vi "MCCMSG Select Multi Clamp.vi"(0 "hMCCmsg":i32, 1 "uDeviceID":u32, 2 "pnError":i32, 5 "uModel":u32, 7 "pszSerialNum":string, 9 "uCOMPortID":u32, 11 "error in (no error)":errorcluster, 12 "uChannelID":u32) -> (4 "pnError out":i32, 6 "function return":i32, 8 "pszSerialNum out":string, 15 "error out":errorcluster)   [LabVIEW 2012, in "MultiClamp 700B Controls.lvlib" / "AxMultiClampMsg.lvlib"]
doc: "AXMCCMSG BOOL WINAPI MCCMSG_SelectMultiClamp(HMCCMSG hMCCmsg, UINT uModel, char *pszSerialNum, UINT uCOMPortID, UINT uDeviceID, UINT uChannelID, int *pnError);"
uses:
  AxMultiClampMsg.lvlib
  AxMultiClampMsg.dll
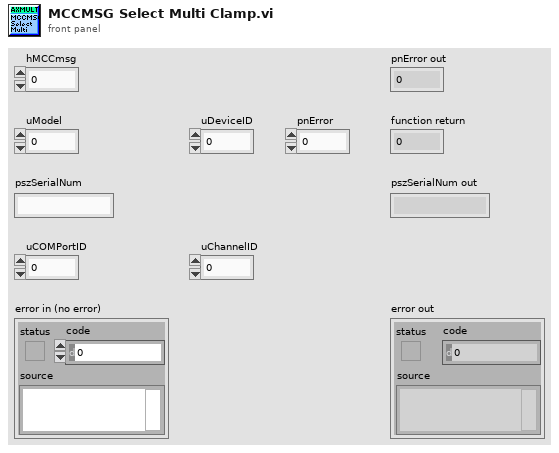
[diagram p1: front panel]
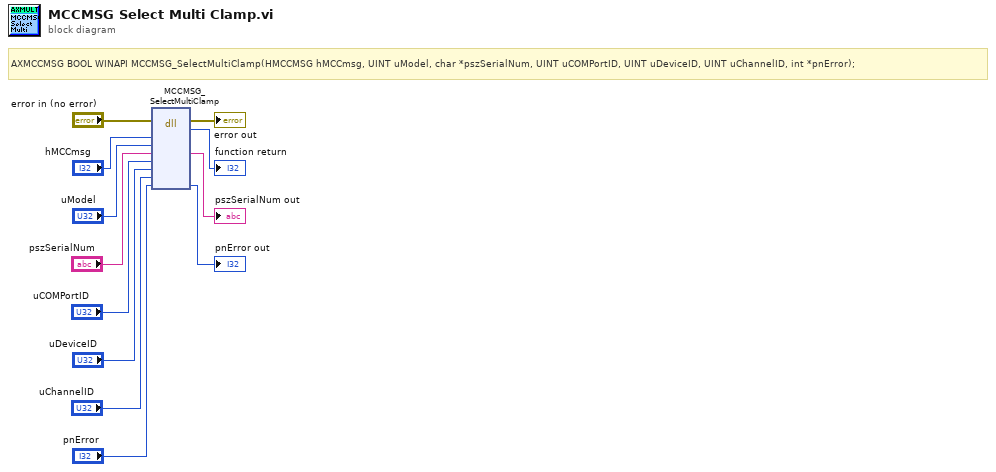
[diagram p0: block diagram]
diagram:
  # "AXMCCMSG BOOL WINAPI MCCMSG_SelectMultiClamp(HMCCMSG hMCCmsg, UINT uModel, char *pszSerialNum, UINT uCOMPortID, UINT uDeviceID, UINT uChannelID, int *pnError);"
  n1 = dll-call lib="C:/Users/Southampton/Desktop/Rita/Multiclamp 700B VIs/AxMultiClampMsg/AxMultiClampMsg.*" fn="MCCMSG_SelectMultiClamp"(error in="error in (no error)", "hMCCmsg"="hMCCmsg", "uModel"="uModel", "pszSerialNum"="pszSerialNum", "uCOMPortID"="uCOMPortID", "uDeviceID"="uDeviceID", "uChannelID"="uChannelID", "pnError"="pnError") -> (error out=→"error out":errorcluster, →"function return":i32, "pszSerialNum"=→"pszSerialNum out":string, "pnError"=→"pnError out":i32)  [unwired: 7 in, 1 out]
